vi "DEMO_CameraManager.vi"() -> ()   [LabVIEW 2017, in "PlayNitrideCameraComponet1010_4.lvlib"]
uses:
  <userlib>/PlayNitrideCameraComponet1010_4/PlayNitrideCameraComponet1010_4.lvlib
panel:
  out "Spend Time(ms)":u32
  out "error out":errorcluster
  in  "Select Command":string(combo)
  out "Camera Manage UI":enum32{"Data In", "Data Out"}(tab) caption="Camera Manage Data Visualize"
  in  "Camera Manager Data":T2={"Camera Index"=0.0, "Exposure Time"=2800.0, "Image"=refnum, "Save Img Path"=path "C:/Users/MyUser/Pictures", "error out"={"status"=FALSE, "code"=0, "source"=""}, "Specific Parameter"={"Parameter Name"="", "Parameter Value"=""}, "Image Info"={"Height"=0.0, "Width"=0.0, "Channels"=0.0}}
  out "Camera Manager Data Output":T2={"Camera Index"=0.0, "Exposure Time"=2800.0, "Image"=refnum, "Save Img Path"=path "C:/Users/MyUser/Pictures", "error out"={"status"=FALSE, "code"=0, "source"=""}, "Specific Parameter"={"Parameter Name"="", "Parameter Value"=""}, "Image Info"={"Height"=0.0, "Width"=0.0, "Channels"=0.0}}
  out "Image View":T1(plugin-control)
  out "Queue out":refnum<queue>
  out "save img path":path
  in  "Pic Path":path=path "C:/Users/DavidHsu/OneDrive - PlayNitride/L0_230912/pic/key_pic/20x_2040_rf_k31l.bmp"
  in  "Cluster In":T3={"Camera Mode"=FALSE, "顯示準星"=FALSE, "準星顏色"=65469}
  in  "Save Setting":T4
  in  "Queue in":refnum<queue>
  # "Extra Param"
  # "Extra Output"
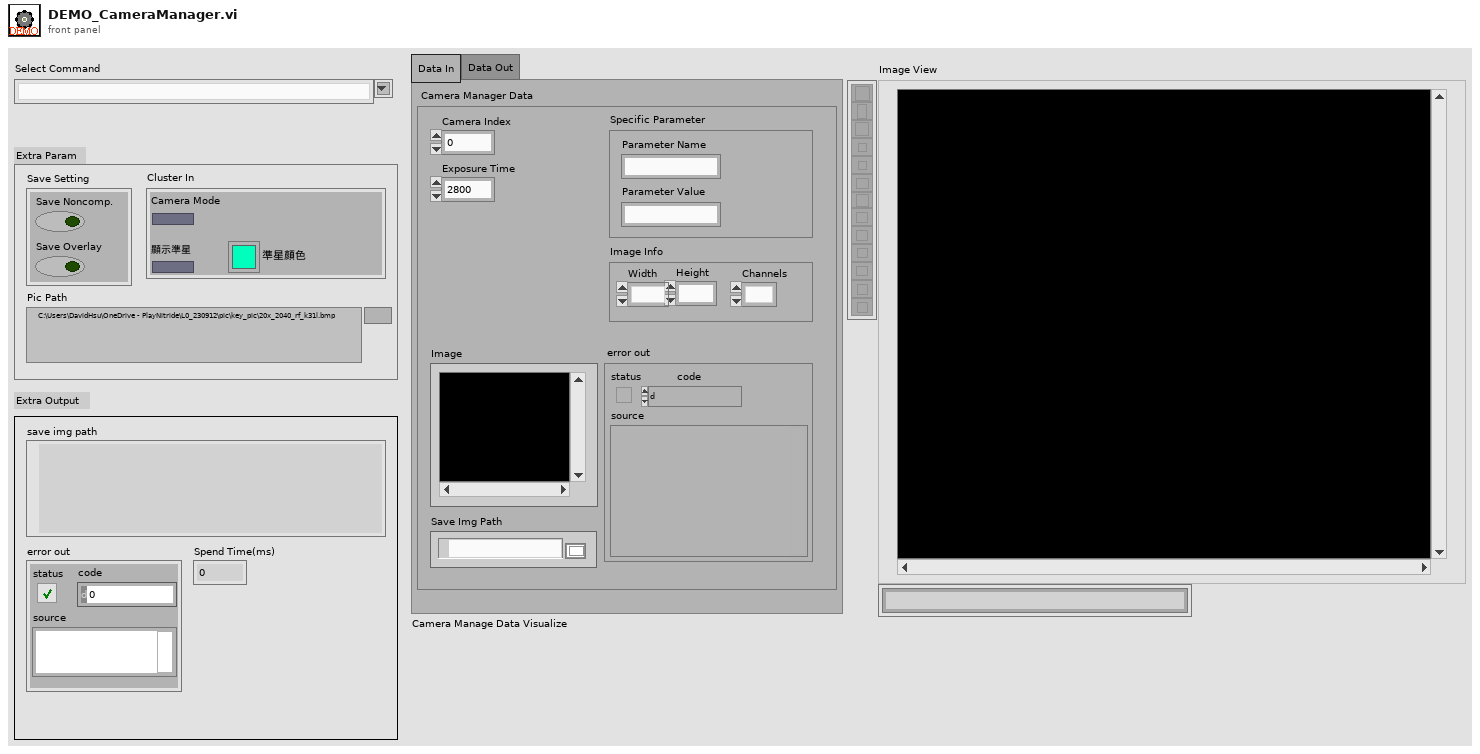
[diagram p1: front panel]
types:
  T1 = typedef "IMAQ Image.ctl" = refnum<image>
  T2 = cluster{"Camera Index":dbl, "Exposure Time":dbl, "Image":T1, "Save Img Path":path, "error out":errorcluster, "Specific Parameter":cluster{"Parameter Name":string, "Parameter Value":string}, "Image Info":cluster{"Height":dbl, "Width":dbl, "Channels":dbl}}
  T3 = cluster{"Camera Mode":bool, "顯示準星":bool, "準星顏色":u32}
  T4 = cluster{"Save Noncomp.":bool, "Save Overlay":bool}
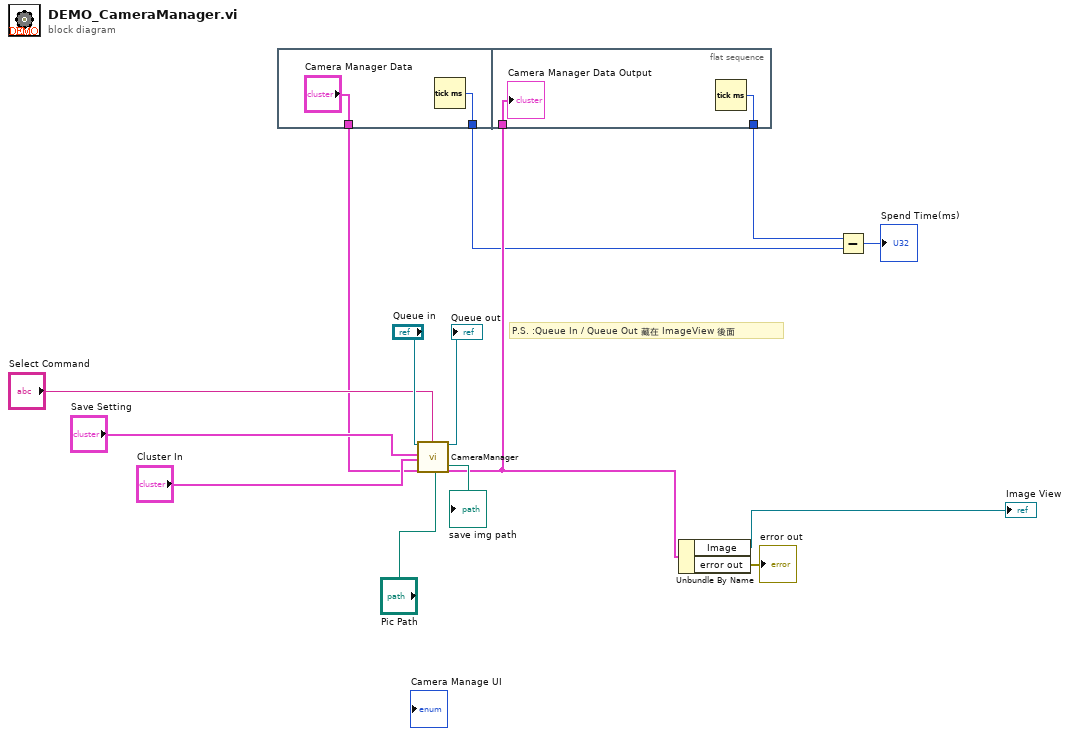
[diagram p0: block diagram]
diagram:
  # "P.S. :Queue In / Queue Out 藏在 ImageView 後面"
  n1 = flat-sequence {
    tunnel: ["Camera Manager Data"] -> w5
    tunnel: [w15] -> w1
    tunnel: w4 -> [w18]
    tunnel: [w17] -> w2
    frame #0 {
      n2 = Tick Count (ms)() -> (millisecond timer value=w15:u32)
    }
    frame #1 {
      n3 = Tick Count (ms)() -> (millisecond timer value=w17:u32)
      "Camera Manager Data Output" <- w18
    }
  }
  n4 = call <userlib>:"CameraManager.vi"("Queue in"="Queue in", "Save Setting"="Save Setting", "Cluster In"="Cluster In", "Camera Manager Data"=w5, "Select Case"="Select Command", "Pic Path"="Pic Path") -> ("save img path"=→"save img path":path, "Queue out"=→"Queue out":refnum<queue>, "Camera Manager Data Output"=w4:T2)  [unwired: 8 in, 3 out]
  n5 = Unbundle By Name(w4) -> ("Image"=→"Image View":T1, "error out"=→"error out":errorcluster)
  n6 = Subtract(x=w2, y=w1) -> (x-y=→"Spend Time(ms)":u32)
